vi "Configuration.vi"(8 "error in (no error)":errorcluster, 9 "Source Delay (Sec)":dbl, 10 "Load SMU Channel":string, 11 "IVI Refnum in":refnum<k15>) -> (0 "error out":errorcluster, 2 "Current Measurement":dbl, 3 "Voltage Measurement":dbl)   [LabVIEW 2021]
uses:
  <instrlib>/niDCPower/nidcpower.llb/niDCPower Wait For Event - Event.ctl
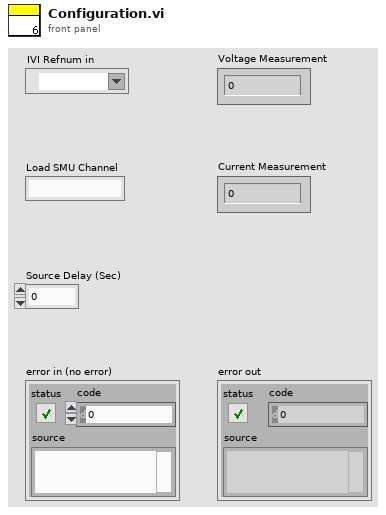
[diagram p1: front panel]
types:
  T1 = typedef "niDCPower Wait For Event - Event.ctl" = i32
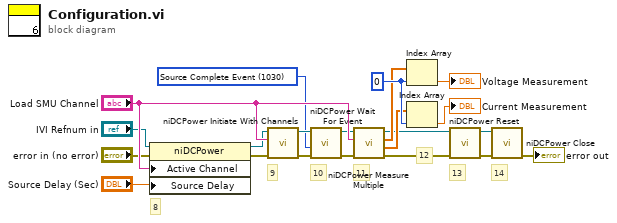
[diagram p0: block diagram]
diagram:
  w15 = T1 1030 items=["Source Complete Event"=1030, "Measure Complete Event"=1031, "Sequence Iteration Complete Event"=1032, "Sequence Engine Done Event"=1033] ("event")
  w7 = 0 ("index")
  # "14"
  # "8"
  # "11"
  # "10"
  # "12"
  # "13"
  # "9"
  n1 = property class="niDCPower"(reference="IVI Refnum in", error in="error in (no error)", "Active Channel"="Load SMU Channel", "Source Delay"="Source Delay (Sec)") -> (reference out=w17:refnum<k15>, error out=w20:errorcluster)
  n2 = call <instrlib>:"niDCPower Initiate With Channels.vi"("error in (no error)"=w20, "channel name"="Load SMU Channel", "instrument handle"=w17) -> ("error out"=w18:errorcluster, "instrument handle out"=w19:refnum<k15>)  [unwired: 7 in]
  n3 = call <instrlib>:"niDCPower Wait For Event.vi"("error in (no error)"=w18, "event"=w15, "instrument handle"=w19) -> ("error out"=w14:errorcluster, "instrument handle out"=w13:refnum<k15>)  [unwired: 1 in, 6 out]
  n4 = call <instrlib>:"niDCPower Measure Multiple.vi"("error in (no error)"=w14, "channel name"="Load SMU Channel", "instrument handle"=w13) -> ("error out"=w4:errorcluster, "current measurements"=w6:dbl[], "voltage measurements"=w5:dbl[], "instrument handle out"=w3:refnum<k15>)  [unwired: 5 out]
  n5 = Index Array(array=w5, index=w7) -> (element=→"Voltage Measurement":dbl)
  n6 = Index Array(array=w6, index=w7) -> (element=→"Current Measurement":dbl)
  n7 = call <instrlib>:"niDCPower Reset.vi"("error in (no error)"=w4, "instrument handle"=w3) -> ("error out"=w2:errorcluster, "instrument handle out"=w1:refnum<k15>)  [unwired: 2 in, 6 out]
  n8 = call <instrlib>:"niDCPower Close.vi"("error in (no error)"=w2, "instrument handle"=w1) -> ("error out"=→"error out":errorcluster)  [unwired: 9 out]
